vi "nav waypoint info.vi"(11 "step":i32) -> (0 "target y":i32, 1 "target x":i32, 2 "load":i32, 3 "stacking height":dbl, 4 "steps":i32)   [LabVIEW 2014]
uses:
  <vilib>/Rock Robotics/Network Tables/SD Read Boolean Array.vi
  Robot Global Data.vi
panel:
  out "Button States":bool[](array[boolean])
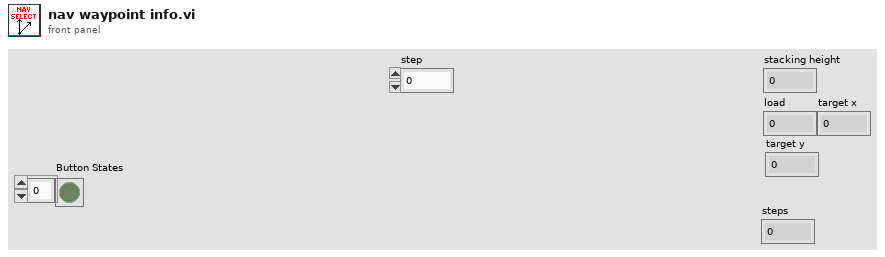
[diagram p1: front panel]
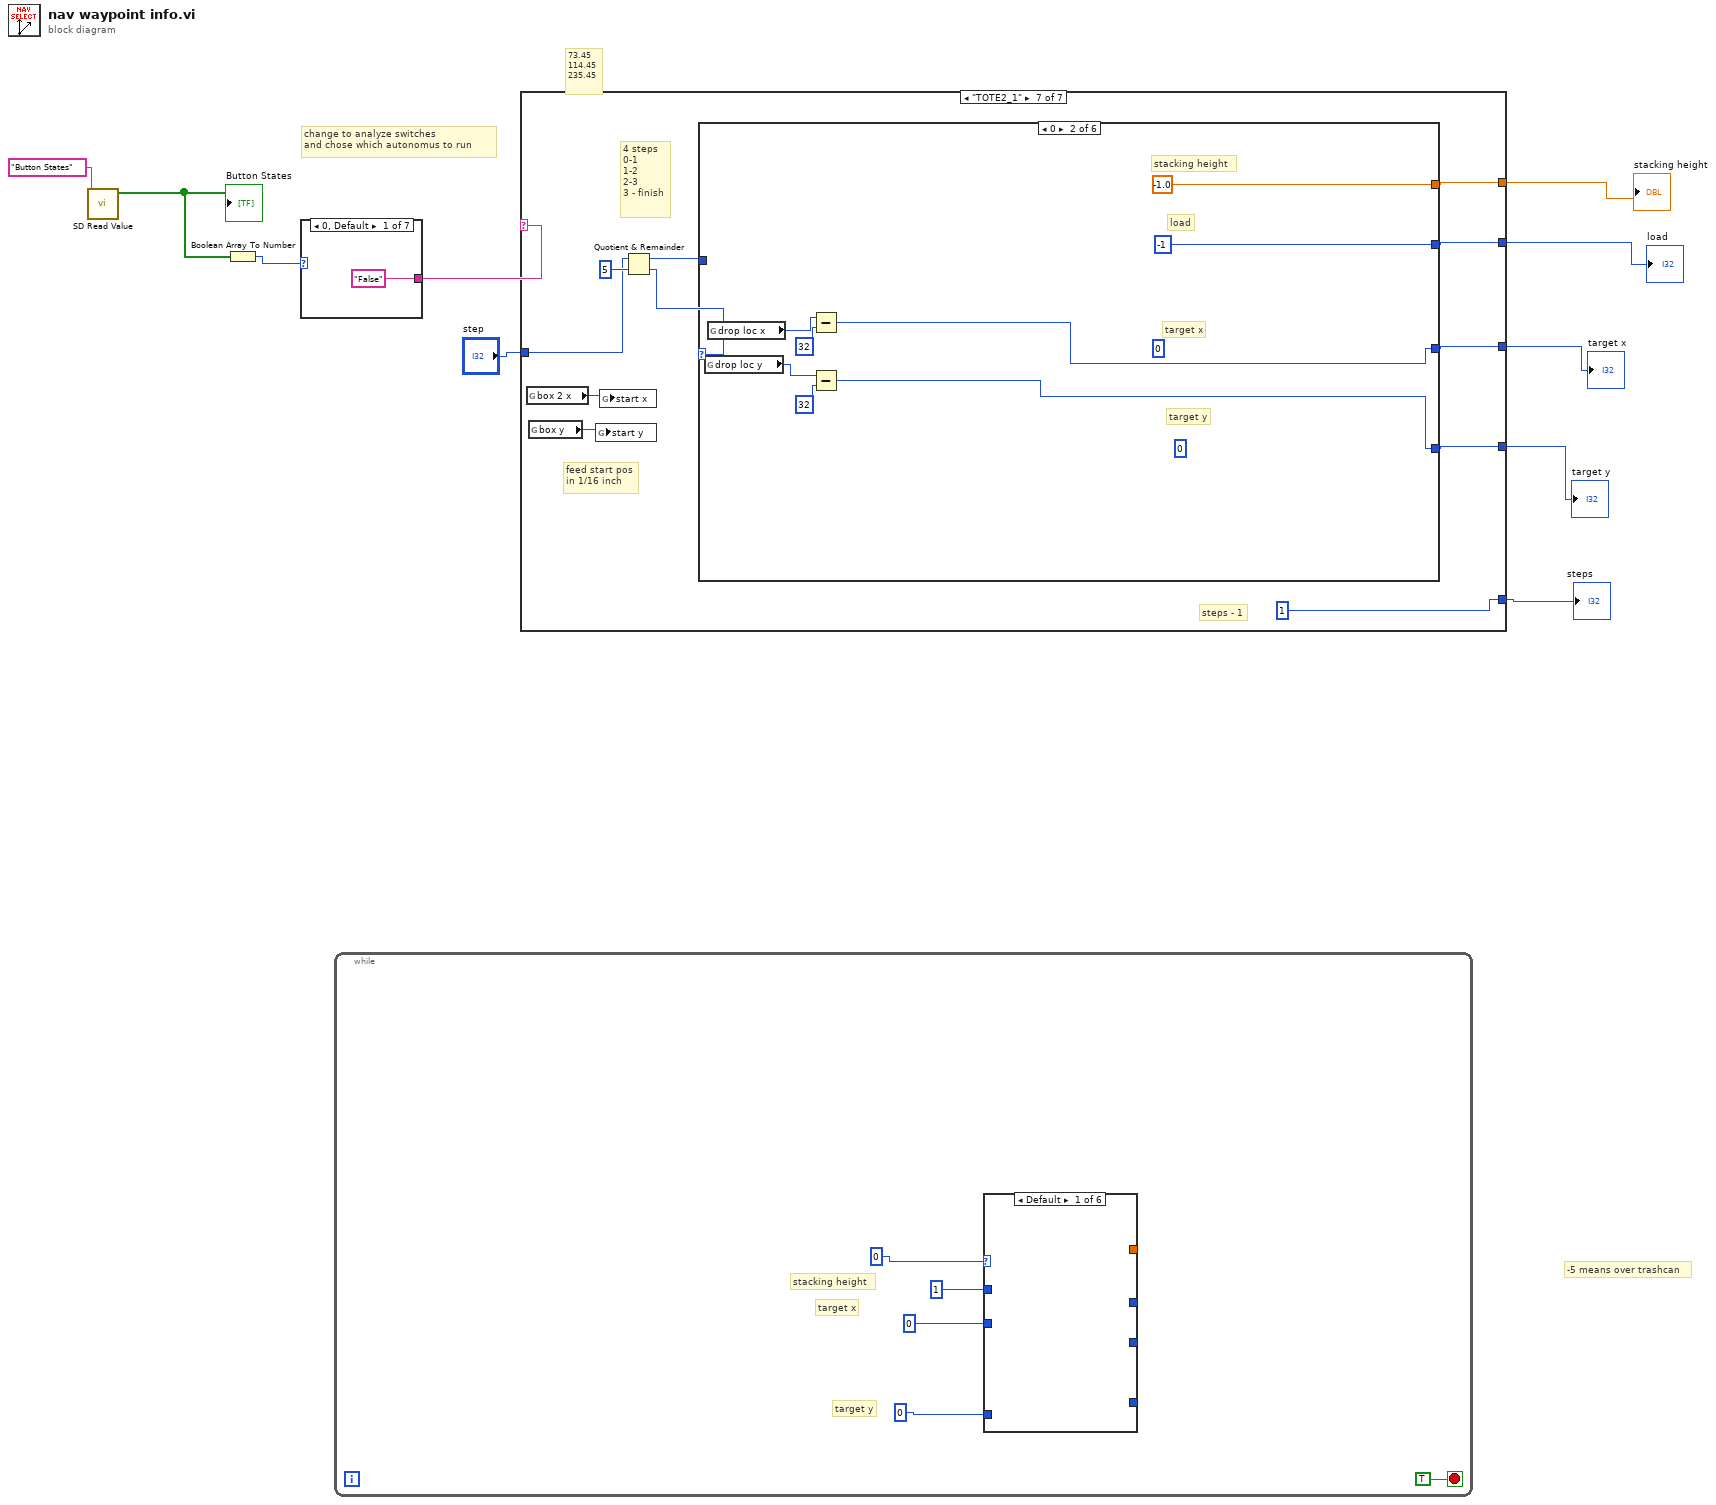
[diagram p0: block diagram]
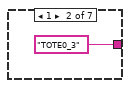
[diagram p2: hidden frame]
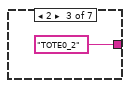
[diagram p3: hidden frame]
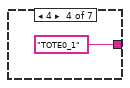
[diagram p4: hidden frame]
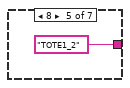
[diagram p5: hidden frame]
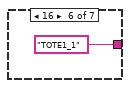
[diagram p6: hidden frame]
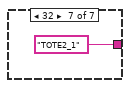
[diagram p7: hidden frame]
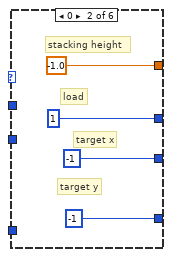
[diagram p8: hidden frame]
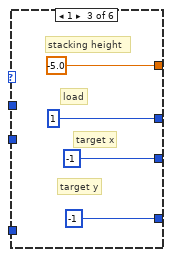
[diagram p9: hidden frame]
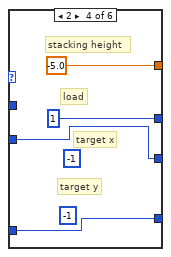
[diagram p10: hidden frame]
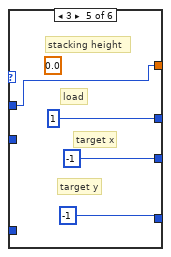
[diagram p11: hidden frame]
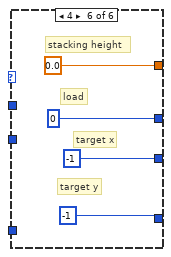
[diagram p12: hidden frame]
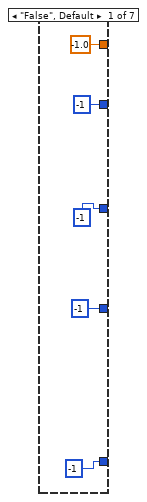
[diagram p13: hidden frame]
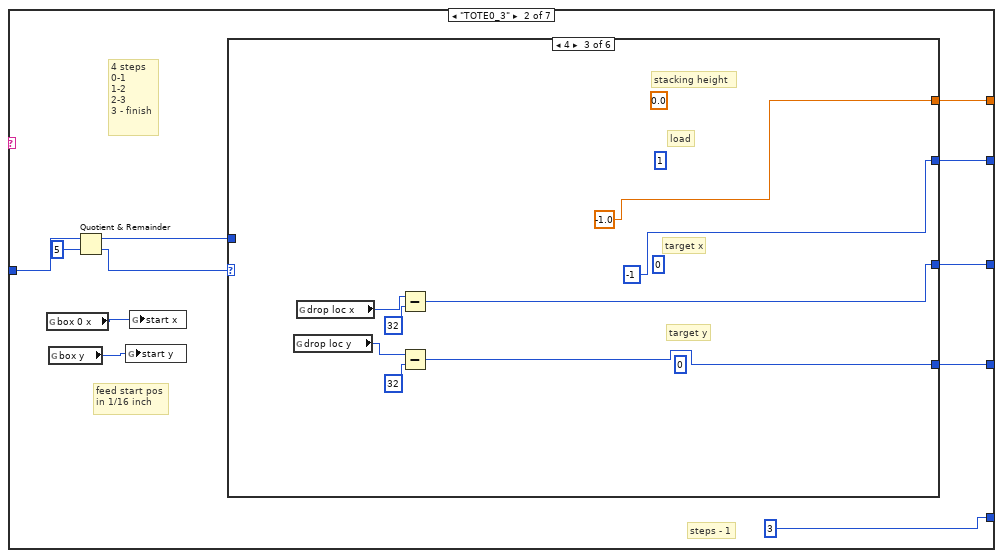
[diagram p14: hidden frame]
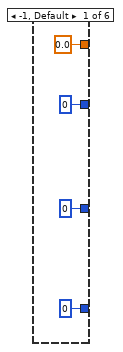
[diagram p15: hidden frame]
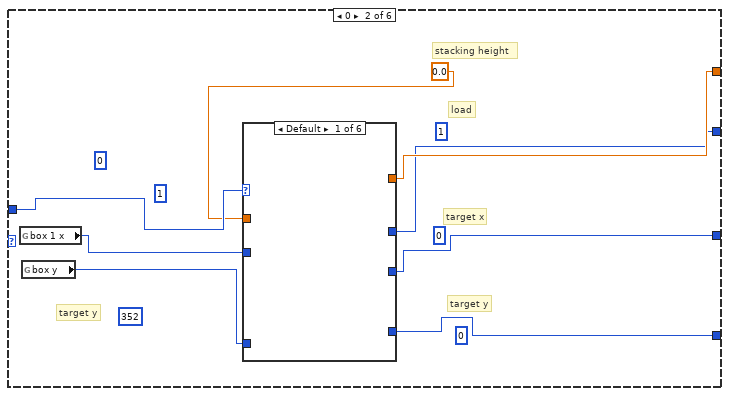
[diagram p16: hidden frame]
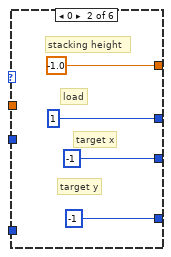
[diagram p17: hidden frame]
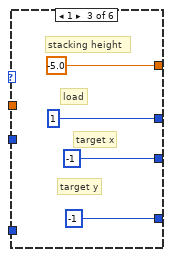
[diagram p18: hidden frame]
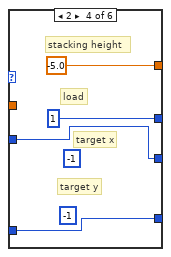
[diagram p19: hidden frame]
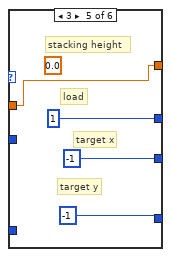
[diagram p20: hidden frame]
diagram:
  # "73.45\n114.45\n235.45"
  # "-5 means over trashcan"
  # "change to analyze switches\nand chose which autonomus to run"
  n1 = call-poly <vilib>:"SD Read Value.vi"("Name"="Button States") -> ("Boolean Array"=w3:bool[])  [unwired: 8 in, 2 out]
  "Button States" <- w3
  n2 = Boolean Array To Number(Boolean array=w3) -> (number=w2:u32)
  n3 = case shown="0, Default" w2 {
    tunnel: ["False" "TOTE0_3" "TOTE0_2" "TOTE0_1" "TOTE1_2" "TOTE1_1" "TOTE2_1"] -> w1
    frame 0, Default {
    }
    frame 1 {
    }
    frame 2 {
    }
    frame 4 {
    }
    frame 8 {
    }
    frame 16 {
    }
    frame 32 {
    }
  }
  n4 = while {
    stop <- TRUE stop-if-true
    # "target y"
    # "target x"
    # "stacking height"
    n5 = case shown="Default" 0 {
      tunnel: [_ -1.0 -5.0 -5.0 w35 0.0] -> _
      tunnel: [_ 1 1 1 1 0] -> _
      tunnel: [_ -1 -1 w34 -1 -1] -> _
      tunnel: [_ -1 -1 w33 -1 -1] -> _
      tunnel: 0 -> [_ _ _ w34 _ _]
      tunnel: 0 -> [_ _ _ w33 _ _]
      tunnel: 1 -> [_ _ _ _ w35 _]
      frame Default {
      }
      frame 0 {
        # "target y"
        # "target x"
        # "load"
        # "stacking height"
      }
      frame 1 {
        # "target y"
        # "target x"
        # "load"
        # "stacking height"
      }
      frame 2 {
        (unwired) -1
        (unwired) -1
        # "target y"
        # "target x"
        # "load"
        # "stacking height"
      }
      frame 3 {
        (unwired) 0.0
        # "target y"
        # "target x"
        # "load"
        # "stacking height"
      }
      frame 4 {
        # "target y"
        # "target x"
        # "load"
        # "stacking height"
      }
    }
  }
  n6 = case shown="\"TOTE2_1\"" w1 {
    tunnel: "step" -> [_ w53 w186 w322 w455 w596 w726]
    tunnel: [-1.0 w58 w193 w328 w463 w590 w732] -> w9
    tunnel: [-1 w57 w192 w327 w462 w591 w731] -> w8
    tunnel: [-1 w56 w191 w326 w461 w592 w730] -> w7
    tunnel: [-1 w55 w190 w325 w460 w593 w729] -> w6
    tunnel: [-1 3 2 1 2 1 1] -> w5
    frame "False", Default {
    }
    frame "TOTE0_3" {
      # "feed start pos\nin 1/16 inch"
      # "steps - 1"
      # "4 steps\n0-1\n1-2\n2-3\n3 - finish"
      n7 = global read "Robot Global Data.vi" "box 0 x"() -> (w49:i16)
      n8 = global read "Robot Global Data.vi" "box y"() -> (w48:i16)
      n9 = Quotient & Remainder(x=w53, y=5) -> (x-y*floor(x/y)=w50:i32, floor(x/y)=w51:i32)
      n10 = global write "Robot Global Data.vi" "start y"(w48) -> ()
      n11 = global write "Robot Global Data.vi" "start x"(w49) -> ()
      n12 = case shown="4" w51 {
        tunnel: [0.0 w66 -1.0 w106 w133 w160] -> w58
        tunnel: [0 w65 -1 w103 w132 w159] -> w57
        tunnel: [0 w67 w92 w102 w131 w157] -> w56
        tunnel: [0 w68 w91 w101 w130 w158] -> w55
        tunnel: w50 -> [_ w70 _ w104 w129 w162]
        frame -1, Default {
        }
        frame 0 {
          (unwired) 1
          (unwired) 352
          (unwired) 0
          (unwired) 0
          (unwired) 0
          (unwired) 1
          # "target y"
          # "target y"
          # "target x"
          # "load"
          # "stacking height"
          n13 = global read "Robot Global Data.vi" "box 1 x"() -> (w64:i16)
          n14 = global read "Robot Global Data.vi" "box y"() -> (w63:i16)
          n15 = case shown="Default" w70 {
            tunnel: [_ -1.0 -5.0 -5.0 w83 0.0] -> w66
            tunnel: [_ 1 1 1 1 0] -> w65
            tunnel: [_ -1 -1 w82 -1 -1] -> w67
            tunnel: [_ -1 -1 w81 -1 -1] -> w68
            tunnel: w64 -> [_ _ _ w82 _ _]
            tunnel: w63 -> [_ _ _ w81 _ _]
            tunnel: 0.0 -> [_ _ _ _ w83 _]
            frame Default {
            }
            frame 0 {
              # "target y"
              # "target x"
              # "load"
              # "stacking height"
            }
            frame 1 {
              # "target y"
              # "target x"
              # "load"
              # "stacking height"
            }
            frame 2 {
              (unwired) -1
              (unwired) -1
              # "target y"
              # "target x"
              # "load"
              # "stacking height"
            }
            frame 3 {
              (unwired) 0.0
              # "target y"
              # "target x"
              # "load"
              # "stacking height"
            }
            frame 4 {
              # "target y"
              # "target x"
              # "load"
              # "stacking height"
            }
          }
        }
        frame 4 {
          (unwired) 0
          (unwired) 0
          (unwired) 1
          (unwired) 0.0
          # "target y"
          # "target x"
          # "load"
          # "stacking height"
          n16 = global read "Robot Global Data.vi" "drop loc y"() -> (w93:i16)
          n17 = global read "Robot Global Data.vi" "drop loc x"() -> (w96:i16)
          n18 = Subtract(x=w96, y=i16 32) -> (x-y=w92:i16)
          n19 = Subtract(x=w93, y=i16 32) -> (x-y=w91:i16)
        }
        frame 1 {
          (unwired) 0
          (unwired) 0
          (unwired) 1
          # "target y"
          # "target x"
          # "load"
          # "stacking height inchs"
          n20 = global read "Robot Global Data.vi" "box 2 x"() -> (w99:i16)
          n21 = global read "Robot Global Data.vi" "box y"() -> (w100:i16)
          n22 = case shown="Default" w104 {
            tunnel: [_ -1.0 -5.0 -5.0 w119 0.0] -> w106
            tunnel: [_ 1 1 1 1 0] -> w103
            tunnel: [_ -1 -1 w118 -1 -1] -> w102
            tunnel: [_ -1 -1 w117 -1 -1] -> w101
            tunnel: w99 -> [_ _ _ w118 _ _]
            tunnel: w100 -> [_ _ _ w117 _ _]
            tunnel: 12.1 -> [_ _ _ _ w119 _]
            frame Default {
            }
            frame 0 {
              # "target y"
              # "target x"
              # "load"
              # "stacking height"
            }
            frame 1 {
              # "target y"
              # "target x"
              # "load"
              # "stacking height"
            }
            frame 2 {
              (unwired) -1
              (unwired) -1
              # "target y"
              # "target x"
              # "load"
              # "stacking height"
            }
            frame 3 {
              (unwired) 0.0
              # "target y"
              # "target x"
              # "load"
              # "stacking height"
            }
            frame 4 {
              # "target y"
              # "target x"
              # "load"
              # "stacking height"
            }
          }
        }
        frame 2 {
          (unwired) 0
          (unwired) 0
          (unwired) 1
          # "to box 3"
          # "target y"
          # "target x"
          # "load"
          # "stacking height inchs"
          n23 = global read "Robot Global Data.vi" "box 2 x"() -> (w128:i16)
          n24 = global read "Robot Global Data.vi" "box y"() -> (w127:i16)
          n25 = case shown="Default" w129 {
            tunnel: [_ -1.0 -5.0 -5.0 w147 0.0] -> w133
            tunnel: [_ 1 1 1 1 0] -> w132
            tunnel: [_ -1 -1 w146 -1 -1] -> w131
            tunnel: [_ -1 -1 w145 -1 -1] -> w130
            tunnel: w128 -> [_ _ _ w146 _ _]
            tunnel: w127 -> [_ _ _ w145 _ _]
            tunnel: 24.2 -> [_ _ _ _ w147 _]
            frame Default {
            }
            frame 0 {
              # "target y"
              # "target x"
              # "load"
              # "stacking height"
            }
            frame 1 {
              # "target y"
              # "target x"
              # "load"
              # "stacking height"
            }
            frame 2 {
              (unwired) -1
              (unwired) -1
              # "target y"
              # "target x"
              # "load"
              # "stacking height"
            }
            frame 3 {
              (unwired) 0.0
              # "target y"
              # "target x"
              # "load"
              # "stacking height"
            }
            frame 4 {
              # "target y"
              # "target x"
              # "load"
              # "stacking height"
            }
          }
        }
        frame 3 {
          (unwired) 0
          (unwired) 0
          (unwired) 0
          # "steps"
          # "target y"
          # "target x"
          # "load"
          # "stacking height inchs"
          n26 = global read "Robot Global Data.vi" "drop loc y"() -> (w155:i16)
          n27 = global read "Robot Global Data.vi" "drop loc x"() -> (w156:i16)
          n28 = case shown="4" w162 {
            tunnel: [_ -1.0 -5.0 -5.0 w175 0.0] -> w160
            tunnel: [_ 1 1 1 1 0] -> w159
            tunnel: [_ -1 -1 w174 -1 -1] -> w157
            tunnel: [_ -1 -1 w173 -1 -1] -> w158
            tunnel: w156 -> [_ _ _ w174 _ _]
            tunnel: w155 -> [_ _ _ w173 _ _]
            tunnel: 4.0 -> [_ _ _ _ w175 _]
            frame Default {
            }
            frame 0 {
              # "target y"
              # "target x"
              # "load"
              # "stacking height"
            }
            frame 1 {
              # "target y"
              # "target x"
              # "load"
              # "stacking height"
            }
            frame 2 {
              (unwired) -1
              (unwired) -1
              # "target y"
              # "target x"
              # "load"
              # "stacking height"
            }
            frame 3 {
              (unwired) 0.0
              # "target y"
              # "target x"
              # "load"
              # "stacking height"
            }
            frame 4 {
              # "target y"
              # "target x"
              # "load"
              # "stacking height"
            }
          }
        }
      }
    }
    frame "TOTE0_2" {
      # "feed start pos\nin 1/16 inch"
      # "steps - 1"
      # "4 steps\n0-1\n1-2\n2-3\n3 - finish"
      n29 = global read "Robot Global Data.vi" "box 0 x"() -> (w183:i16)
      n30 = global read "Robot Global Data.vi" "box y"() -> (w184:i16)
      n31 = Quotient & Remainder(x=w186, y=5) -> (x-y*floor(x/y)=w187:i32, floor(x/y)=w185:i32)
      n32 = global write "Robot Global Data.vi" "start y"(w184) -> ()
      n33 = global write "Robot Global Data.vi" "start x"(w183) -> ()
      n34 = case shown="2" w185 {
        tunnel: [0.0 w204 w232 w260 -1.0 w295] -> w193
        tunnel: [0 w203 w231 w259 -1 w294] -> w192
        tunnel: [0 w201 w230 w258 w284 w291] -> w191
        tunnel: [0 w202 w229 w257 w285 w290] -> w190
        tunnel: w187 -> [_ w200 w228 w256 _ w296]
        frame -1, Default {
        }
        frame 0 {
          (unwired) 0
          (unwired) 0
          (unwired) 0
          # "target y"
          # "target x"
          # "load"
          # "stacking height"
          n35 = global read "Robot Global Data.vi" "box 2 x"() -> (w199:i16)
          n36 = global read "Robot Global Data.vi" "box y"() -> (w198:i16)
          n37 = case shown="Default" w200 {
            tunnel: [_ -1.0 -5.0 -5.0 w218 0.0] -> w204
            tunnel: [_ 1 1 1 1 0] -> w203
            tunnel: [_ -1 -1 w217 -1 -1] -> w201
            tunnel: [_ -1 -1 w216 -1 -1] -> w202
            tunnel: w199 -> [_ _ _ w217 _ _]
            tunnel: w198 -> [_ _ _ w216 _ _]
            tunnel: 0.0 -> [_ _ _ _ w218 _]
            frame Default {
            }
            frame 0 {
              # "target y"
              # "target x"
              # "load"
              # "stacking height"
            }
            frame 1 {
              # "target y"
              # "target x"
              # "load"
              # "stacking height"
            }
            frame 2 {
              (unwired) -1
              (unwired) -1
              # "target y"
              # "target x"
              # "load"
              # "stacking height"
            }
            frame 3 {
              (unwired) 0.0
              # "target y"
              # "target x"
              # "load"
              # "stacking height"
            }
            frame 4 {
              # "target y"
              # "target x"
              # "load"
              # "stacking height"
            }
          }
        }
        frame 4 {
          (unwired) 0
          (unwired) 0
          (unwired) 1
          # "target y"
          # "target x"
          # "load"
          # "stacking height"
          n38 = global read "Robot Global Data.vi" "box 0 x"() -> (w227:i16)
          n39 = global read "Robot Global Data.vi" "box y"() -> (w226:i16)
          n40 = case shown="Default" w228 {
            tunnel: [_ -1.0 -5.0 -5.0 w246 0.0] -> w232
            tunnel: [_ 1 1 1 1 0] -> w231
            tunnel: [_ -1 -1 w245 -1 -1] -> w230
            tunnel: [_ -1 -1 w244 -1 -1] -> w229
            tunnel: w227 -> [_ _ _ w245 _ _]
            tunnel: w226 -> [_ _ _ w244 _ _]
            tunnel: 0.0 -> [_ _ _ _ w246 _]
            frame Default {
            }
            frame 0 {
              # "target y"
              # "target x"
              # "load"
              # "stacking height"
            }
            frame 1 {
              # "target y"
              # "target x"
              # "load"
              # "stacking height"
            }
            frame 2 {
              (unwired) -1
              (unwired) -1
              # "target y"
              # "target x"
              # "load"
              # "stacking height"
            }
            frame 3 {
              (unwired) 0.0
              # "target y"
              # "target x"
              # "load"
              # "stacking height"
            }
            frame 4 {
              # "target y"
              # "target x"
              # "load"
              # "stacking height"
            }
          }
        }
        frame 1 {
          (unwired) 0
          (unwired) 0
          (unwired) 1
          # "target y"
          # "target x"
          # "load"
          # "stacking height inchs"
          n41 = global read "Robot Global Data.vi" "drop loc y"() -> (w254:i16)
          n42 = global read "Robot Global Data.vi" "drop loc x"() -> (w255:i16)
          n43 = case shown="Default" w256 {
            tunnel: [_ -1.0 -5.0 -5.0 w274 0.0] -> w260
            tunnel: [_ 1 1 1 1 0] -> w259
            tunnel: [_ -1 -1 w273 -1 -1] -> w258
            tunnel: [_ -1 -1 w272 -1 -1] -> w257
            tunnel: w255 -> [_ _ _ w273 _ _]
            tunnel: w254 -> [_ _ _ w272 _ _]
            tunnel: 12.1 -> [_ _ _ _ w274 _]
            frame Default {
            }
            frame 0 {
              # "target y"
              # "target x"
              # "load"
              # "stacking height"
            }
            frame 1 {
              # "target y"
              # "target x"
              # "load"
              # "stacking height"
            }
            frame 2 {
              (unwired) -1
              (unwired) -1
              # "target y"
              # "target x"
              # "load"
              # "stacking height"
            }
            frame 3 {
              (unwired) 0.0
              # "target y"
              # "target x"
              # "load"
              # "stacking height"
            }
            frame 4 {
              # "target y"
              # "target x"
              # "load"
              # "stacking height"
            }
          }
        }
        frame 2 {
          (unwired) 0
          (unwired) 0
          # "target y"
          # "target x"
          # "load"
          # "stacking height inchs"
          n44 = global read "Robot Global Data.vi" "drop loc y"() -> (w286:i16)
          n45 = global read "Robot Global Data.vi" "drop loc x"() -> (w289:i16)
          n46 = Subtract(x=w289, y=i16 32) -> (x-y=w284:i16)
          n47 = Subtract(x=w286, y=i16 32) -> (x-y=w285:i16)
        }
        frame 3 {
          (unwired) 0
          # "steps"
          # "target y"
          # "target x"
          # "load"
          # "stacking height inchs"
          n48 = case shown="Default" w296 {
            tunnel: [_ -1.0 -5.0 -5.0 w310 0.0] -> w295
            tunnel: [_ 1 1 1 1 0] -> w294
            tunnel: [_ -1 -1 w309 -1 -1] -> w291
            tunnel: [_ -1 -1 w308 -1 -1] -> w290
            tunnel: 0 -> [_ _ _ w309 _ _]
            tunnel: 0 -> [_ _ _ w308 _ _]
            tunnel: 4.0 -> [_ _ _ _ w310 _]
            frame Default {
            }
            frame 0 {
              # "target y"
              # "target x"
              # "load"
              # "stacking height"
            }
            frame 1 {
              # "target y"
              # "target x"
              # "load"
              # "stacking height"
            }
            frame 2 {
              (unwired) -1
              (unwired) -1
              # "target y"
              # "target x"
              # "load"
              # "stacking height"
            }
            frame 3 {
              (unwired) 0.0
              # "target y"
              # "target x"
              # "load"
              # "stacking height"
            }
            frame 4 {
              # "target y"
              # "target x"
              # "load"
              # "stacking height"
            }
          }
        }
      }
    }
    frame "TOTE0_1" {
      # "feed start pos\nin 1/16 inch"
      # "steps - 1"
      # "4 steps\n0-1\n1-2\n2-3\n3 - finish"
      n49 = global read "Robot Global Data.vi" "box 0 x"() -> (w319:i16)
      n50 = global read "Robot Global Data.vi" "box y"() -> (w318:i16)
      n51 = global write "Robot Global Data.vi" "start y"(w318) -> ()
      n52 = global write "Robot Global Data.vi" "start x"(w319) -> ()
      n53 = Quotient & Remainder(x=w322, y=5) -> (x-y*floor(x/y)=w321:i32, floor(x/y)=w320:i32)
      n54 = case shown="1" w320 {
        tunnel: [0.0 w339 w368 -1.0 w402 w432] -> w328
        tunnel: [0 w338 w366 -1 w401 w431] -> w327
        tunnel: [0 w337 w363 w392 w398 w428] -> w326
        tunnel: [0 w336 w362 w391 w397 w427] -> w325
        tunnel: w321 -> [_ w335 w361 _ w403 w425]
        frame -1, Default {
        }
        frame 0 {
          (unwired) 0
          (unwired) 0
          (unwired) 1
          # "target y"
          # "target x"
          # "load"
          # "stacking height"
          n55 = global read "Robot Global Data.vi" "drop loc y"() -> (w333:i16)
          n56 = global read "Robot Global Data.vi" "drop loc x"() -> (w334:i16)
          n57 = case shown="Default" w335 {
            tunnel: [_ -1.0 -5.0 -5.0 w353 0.0] -> w339
            tunnel: [_ 1 1 1 1 0] -> w338
            tunnel: [_ -1 -1 w352 -1 -1] -> w337
            tunnel: [_ -1 -1 w351 -1 -1] -> w336
            tunnel: w334 -> [_ _ _ w352 _ _]
            tunnel: w333 -> [_ _ _ w351 _ _]
            tunnel: 0.0 -> [_ _ _ _ w353 _]
            frame Default {
            }
            frame 0 {
              # "target y"
              # "target x"
              # "load"
              # "stacking height"
            }
            frame 1 {
              # "target y"
              # "target x"
              # "load"
              # "stacking height"
            }
            frame 2 {
              (unwired) -1
              (unwired) -1
              # "target y"
              # "target x"
              # "load"
              # "stacking height"
            }
            frame 3 {
              (unwired) 0.0
              # "target y"
              # "target x"
              # "load"
              # "stacking height"
            }
            frame 4 {
              # "target y"
              # "target x"
              # "load"
              # "stacking height"
            }
          }
        }
        frame 4 {
          (unwired) 1
          # "target y"
          # "target x"
          # "load"
          # "stacking height"
          n58 = case shown="Default" w361 {
            tunnel: [_ -1.0 -5.0 -5.0 w381 0.0] -> w368
            tunnel: [_ 1 1 1 1 0] -> w366
            tunnel: [_ -1 -1 w380 -1 -1] -> w363
            tunnel: [_ -1 -1 w379 -1 -1] -> w362
            tunnel: 0 -> [_ _ _ w380 _ _]
            tunnel: 0 -> [_ _ _ w379 _ _]
            tunnel: 0.0 -> [_ _ _ _ w381 _]
            frame Default {
            }
            frame 0 {
              # "target y"
              # "target x"
              # "load"
              # "stacking height"
            }
            frame 1 {
              # "target y"
              # "target x"
              # "load"
              # "stacking height"
            }
            frame 2 {
              (unwired) -1
              (unwired) -1
              # "target y"
              # "target x"
              # "load"
              # "stacking height"
            }
            frame 3 {
              (unwired) 0.0
              # "target y"
              # "target x"
              # "load"
              # "stacking height"
            }
            frame 4 {
              # "target y"
              # "target x"
              # "load"
              # "stacking height"
            }
          }
        }
        frame 1 {
          (unwired) 0
          (unwired) 0
          # "target y"
          # "target x"
          # "load"
          # "stacking height inchs"
          n59 = global read "Robot Global Data.vi" "drop loc y"() -> (w393:i16)
          n60 = global read "Robot Global Data.vi" "drop loc x"() -> (w396:i16)
          n61 = Subtract(x=w396, y=i16 32) -> (x-y=w392:i16)
          n62 = Subtract(x=w393, y=i16 32) -> (x-y=w391:i16)
        }
        frame 2 {
          (unwired) 1
          # "target y"
          # "target x"
          # "load"
          # "stacking height inchs"
          n63 = case shown="Default" w403 {
            tunnel: [_ -1.0 -5.0 -5.0 w417 0.0] -> w402
            tunnel: [_ 1 1 1 1 0] -> w401
            tunnel: [_ -1 -1 w416 -1 -1] -> w398
            tunnel: [_ -1 -1 w415 -1 -1] -> w397
            tunnel: 0 -> [_ _ _ w416 _ _]
            tunnel: 0 -> [_ _ _ w415 _ _]
            tunnel: 24.2 -> [_ _ _ _ w417 _]
            frame Default {
            }
            frame 0 {
              # "target y"
              # "target x"
              # "load"
              # "stacking height"
            }
            frame 1 {
              # "target y"
              # "target x"
              # "load"
              # "stacking height"
            }
            frame 2 {
              (unwired) -1
              (unwired) -1
              # "target y"
              # "target x"
              # "load"
              # "stacking height"
            }
            frame 3 {
              (unwired) 0.0
              # "target y"
              # "target x"
              # "load"
              # "stacking height"
            }
            frame 4 {
              # "target y"
              # "target x"
              # "load"
              # "stacking height"
            }
          }
        }
        frame 3 {
          (unwired) 0
          # "steps"
          # "target y"
          # "target x"
          # "load"
          # "stacking height inchs"
          n64 = case shown="Default" w425 {
            tunnel: [_ -1.0 -5.0 -5.0 w445 0.0] -> w432
            tunnel: [_ 1 1 1 1 0] -> w431
            tunnel: [_ -1 -1 w444 -1 -1] -> w428
            tunnel: [_ -1 -1 w443 -1 -1] -> w427
            tunnel: 0 -> [_ _ _ w444 _ _]
            tunnel: 0 -> [_ _ _ w443 _ _]
            tunnel: 4.0 -> [_ _ _ _ w445 _]
            frame Default {
            }
            frame 0 {
              # "target y"
              # "target x"
              # "load"
              # "stacking height"
            }
            frame 1 {
              # "target y"
              # "target x"
              # "load"
              # "stacking height"
            }
            frame 2 {
              (unwired) -1
              (unwired) -1
              # "target y"
              # "target x"
              # "load"
              # "stacking height"
            }
            frame 3 {
              (unwired) 0.0
              # "target y"
              # "target x"
              # "load"
              # "stacking height"
            }
            frame 4 {
              # "target y"
              # "target x"
              # "load"
              # "stacking height"
            }
          }
        }
      }
    }
    frame "TOTE1_2" {
      # "feed start pos\nin 1/16 inch"
      # "steps - 1"
      # "4 steps\n0-1\n1-2\n2-3\n3 - finish"
      n65 = global read "Robot Global Data.vi" "box 1 x"() -> (w454:i16)
      n66 = global read "Robot Global Data.vi" "box y"() -> (w453:i16)
      n67 = Quotient & Remainder(x=w455, y=5) -> (x-y*floor(x/y)=w457:i32, floor(x/y)=w456:i32)
      n68 = global write "Robot Global Data.vi" "start y"(w453) -> ()
      n69 = global write "Robot Global Data.vi" "start x"(w454) -> ()
      n70 = case shown="2" w456 {
        tunnel: [0.0 w473 w501 w529 -1.0 w567] -> w463
        tunnel: [0 w472 w500 w528 -1 w564] -> w462
        tunnel: [0 w471 w497 w526 w555 w561] -> w461
        tunnel: [0 w470 w496 w527 w554 w560] -> w460
        tunnel: w457 -> [_ w475 w502 w530 _ w565]
        frame -1, Default {
        }
        frame 0 {
          (unwired) 0
          (unwired) 0
          (unwired) 1
          # "target y"
          # "target x"
          # "load"
          # "stacking height"
          n71 = global read "Robot Global Data.vi" "box 2 x"() -> (w469:i16)
          n72 = global read "Robot Global Data.vi" "box y"() -> (w468:i16)
          n73 = case shown="Default" w475 {
            tunnel: [_ -1.0 -5.0 -5.0 w488 0.0] -> w473
            tunnel: [_ 1 1 1 1 0] -> w472
            tunnel: [_ -1 -1 w487 -1 -1] -> w471
            tunnel: [_ -1 -1 w486 -1 -1] -> w470
            tunnel: w469 -> [_ _ _ w487 _ _]
            tunnel: w468 -> [_ _ _ w486 _ _]
            tunnel: 0.0 -> [_ _ _ _ w488 _]
            frame Default {
            }
            frame 0 {
              # "target y"
              # "target x"
              # "load"
              # "stacking height"
            }
            frame 1 {
              # "target y"
              # "target x"
              # "load"
              # "stacking height"
            }
            frame 2 {
              (unwired) -1
              (unwired) -1
              # "target y"
              # "target x"
              # "load"
              # "stacking height"
            }
            frame 3 {
              (unwired) 0.0
              # "target y"
              # "target x"
              # "load"
              # "stacking height"
            }
            frame 4 {
              # "target y"
              # "target x"
              # "load"
              # "stacking height"
            }
          }
        }
        frame 4 {
          (unwired) 1
          # "target y"
          # "target x"
          # "load"
          # "stacking height"
          n74 = case shown="Default" w502 {
            tunnel: [_ -1.0 -5.0 -5.0 w516 0.0] -> w501
            tunnel: [_ 1 1 1 1 0] -> w500
            tunnel: [_ -1 -1 w515 -1 -1] -> w497
            tunnel: [_ -1 -1 w514 -1 -1] -> w496
            tunnel: 0 -> [_ _ _ w515 _ _]
            tunnel: 0 -> [_ _ _ w514 _ _]
            tunnel: 0.0 -> [_ _ _ _ w516 _]
            frame Default {
            }
            frame 0 {
              # "target y"
              # "target x"
              # "load"
              # "stacking height"
            }
            frame 1 {
              # "target y"
              # "target x"
              # "load"
              # "stacking height"
            }
            frame 2 {
              (unwired) -1
              (unwired) -1
              # "target y"
              # "target x"
              # "load"
              # "stacking height"
            }
            frame 3 {
              (unwired) 0.0
              # "target y"
              # "target x"
              # "load"
              # "stacking height"
            }
            frame 4 {
              # "target y"
              # "target x"
              # "load"
              # "stacking height"
            }
          }
        }
        frame 1 {
          (unwired) 0
          (unwired) 0
          (unwired) 1
          # "target y"
          # "target x"
          # "load"
          # "stacking height inchs"
          n75 = global read "Robot Global Data.vi" "drop loc y"() -> (w524:i16)
          n76 = global read "Robot Global Data.vi" "drop loc x"() -> (w525:i16)
          n77 = case shown="Default" w530 {
            tunnel: [_ -1.0 -5.0 -5.0 w544 0.0] -> w529
            tunnel: [_ 1 1 1 1 0] -> w528
            tunnel: [_ -1 -1 w543 -1 -1] -> w526
            tunnel: [_ -1 -1 w542 -1 -1] -> w527
            tunnel: w525 -> [_ _ _ w543 _ _]
            tunnel: w524 -> [_ _ _ w542 _ _]
            tunnel: 0.0 -> [_ _ _ _ w544 _]
            frame Default {
            }
            frame 0 {
              # "target y"
              # "target x"
              # "load"
              # "stacking height"
            }
            frame 1 {
              # "target y"
              # "target x"
              # "load"
              # "stacking height"
            }
            frame 2 {
              (unwired) -1
              (unwired) -1
              # "target y"
              # "target x"
              # "load"
              # "stacking height"
            }
            frame 3 {
              (unwired) 0.0
              # "target y"
              # "target x"
              # "load"
              # "stacking height"
            }
            frame 4 {
              # "target y"
              # "target x"
              # "load"
              # "stacking height"
            }
          }
        }
        frame 2 {
          (unwired) 0
          (unwired) 0
          # "target y"
          # "target x"
          # "load"
          # "stacking height inchs"
          n78 = global read "Robot Global Data.vi" "drop loc y"() -> (w556:i16)
          n79 = global read "Robot Global Data.vi" "drop loc x"() -> (w559:i16)
          n80 = Subtract(x=w559, y=i16 32) -> (x-y=w555:i16)
          n81 = Subtract(x=w556, y=i16 32) -> (x-y=w554:i16)
        }
        frame 3 {
          (unwired) 0
          # "steps"
          # "target y"
          # "target x"
          # "load"
          # "stacking height inchs"
          n82 = case shown="Default" w565 {
            tunnel: [_ -1.0 -5.0 -5.0 w580 0.0] -> w567
            tunnel: [_ 1 1 1 1 0] -> w564
            tunnel: [_ -1 -1 w579 -1 -1] -> w561
            tunnel: [_ -1 -1 w578 -1 -1] -> w560
            tunnel: 0 -> [_ _ _ w579 _ _]
            tunnel: 0 -> [_ _ _ w578 _ _]
            tunnel: 4.0 -> [_ _ _ _ w580 _]
            frame Default {
            }
            frame 0 {
              # "target y"
              # "target x"
              # "load"
              # "stacking height"
            }
            frame 1 {
              # "target y"
              # "target x"
              # "load"
              # "stacking height"
            }
            frame 2 {
              (unwired) -1
              (unwired) -1
              # "target y"
              # "target x"
              # "load"
              # "stacking height"
            }
            frame 3 {
              (unwired) 0.0
              # "target y"
              # "target x"
              # "load"
              # "stacking height"
            }
            frame 4 {
              # "target y"
              # "target x"
              # "load"
              # "stacking height"
            }
          }
        }
      }
    }
    frame "TOTE1_1" {
      # "feed start pos\nin 1/16 inch"
      # "steps - 1"
      # "4 steps\n0-1\n1-2\n2-3\n3 - finish"
      n83 = global read "Robot Global Data.vi" "box 1 x"() -> (w589:i16)
      n84 = global read "Robot Global Data.vi" "box y"() -> (w588:i16)
      n85 = global write "Robot Global Data.vi" "start y"(w588) -> ()
      n86 = global write "Robot Global Data.vi" "start x"(w589) -> ()
      n87 = Quotient & Remainder(x=w596, y=5) -> (x-y*floor(x/y)=w595:i32, floor(x/y)=w594:i32)
      n88 = case shown="1" w594 {
        tunnel: [0.0 w609 w637 -1.0 w673 w700] -> w590
        tunnel: [0 w608 w636 -1 w672 w699] -> w591
        tunnel: [0 w606 w635 w662 w669 w696] -> w592
        tunnel: [0 w607 w634 w661 w668 w695] -> w593
        tunnel: w595 -> [_ w605 w633 _ w667 w701]
        frame -1, Default {
        }
        frame 0 {
          (unwired) 0
          (unwired) 0
          (unwired) 0
          # "target y"
          # "target x"
          # "load"
          # "stacking height"
          n89 = global read "Robot Global Data.vi" "drop loc y"() -> (w603:i16)
          n90 = global read "Robot Global Data.vi" "drop loc x"() -> (w604:i16)
          n91 = case shown="Default" w605 {
            tunnel: [_ -1.0 -5.0 -5.0 w623 0.0] -> w609
            tunnel: [_ 1 1 1 1 0] -> w608
            tunnel: [_ -1 -1 w622 -1 -1] -> w606
            tunnel: [_ -1 -1 w621 -1 -1] -> w607
            tunnel: w604 -> [_ _ _ w622 _ _]
            tunnel: w603 -> [_ _ _ w621 _ _]
            tunnel: 0.0 -> [_ _ _ _ w623 _]
            frame Default {
            }
            frame 0 {
              # "target y"
              # "target x"
              # "load"
              # "stacking height"
            }
            frame 1 {
              # "target y"
              # "target x"
              # "load"
              # "stacking height"
            }
            frame 2 {
              (unwired) -1
              (unwired) -1
              # "target y"
              # "target x"
              # "load"
              # "stacking height"
            }
            frame 3 {
              (unwired) 0.0
              # "target y"
              # "target x"
              # "load"
              # "stacking height"
            }
            frame 4 {
              # "target y"
              # "target x"
              # "load"
              # "stacking height"
            }
          }
        }
        frame 4 {
          (unwired) 0
          (unwired) 0
          (unwired) 1
          # "target y"
          # "target x"
          # "load"
          # "stacking height"
          n92 = global read "Robot Global Data.vi" "drop loc y"() -> (w631:i16)
          n93 = global read "Robot Global Data.vi" "drop loc x"() -> (w632:i16)
          n94 = case shown="Default" w633 {
            tunnel: [_ -1.0 -5.0 -5.0 w651 0.0] -> w637
            tunnel: [_ 1 1 1 1 0] -> w636
            tunnel: [_ -1 -1 w650 -1 -1] -> w635
            tunnel: [_ -1 -1 w649 -1 -1] -> w634
            tunnel: w632 -> [_ _ _ w650 _ _]
            tunnel: w631 -> [_ _ _ w649 _ _]
            tunnel: 0.0 -> [_ _ _ _ w651 _]
            frame Default {
            }
            frame 0 {
              # "target y"
              # "target x"
              # "load"
              # "stacking height"
            }
            frame 1 {
              # "target y"
              # "target x"
              # "load"
              # "stacking height"
            }
            frame 2 {
              (unwired) -1
              (unwired) -1
              # "target y"
              # "target x"
              # "load"
              # "stacking height"
            }
            frame 3 {
              (unwired) 0.0
              # "target y"
              # "target x"
              # "load"
              # "stacking height"
            }
            frame 4 {
              # "target y"
              # "target x"
              # "load"
              # "stacking height"
            }
          }
        }
        frame 1 {
          (unwired) 0
          (unwired) 0
          # "target y"
          # "target x"
          # "load"
          # "stacking height inchs"
          n95 = global read "Robot Global Data.vi" "drop loc y"() -> (w663:i16)
          n96 = global read "Robot Global Data.vi" "drop loc x"() -> (w666:i16)
          n97 = Subtract(x=w666, y=i16 32) -> (x-y=w662:i16)
          n98 = Subtract(x=w663, y=i16 32) -> (x-y=w661:i16)
        }
        frame 2 {
          (unwired) 1
          # "target y"
          # "target x"
          # "load"
          # "stacking height inchs"
          n99 = case shown="Default" w667 {
            tunnel: [_ -1.0 -5.0 -5.0 w687 0.0] -> w673
            tunnel: [_ 1 1 1 1 0] -> w672
            tunnel: [_ -1 -1 w686 -1 -1] -> w669
            tunnel: [_ -1 -1 w685 -1 -1] -> w668
            tunnel: 0 -> [_ _ _ w686 _ _]
            tunnel: 0 -> [_ _ _ w685 _ _]
            tunnel: 24.2 -> [_ _ _ _ w687 _]
            frame Default {
            }
            frame 0 {
              # "target y"
              # "target x"
              # "load"
              # "stacking height"
            }
            frame 1 {
              # "target y"
              # "target x"
              # "load"
              # "stacking height"
            }
            frame 2 {
              (unwired) -1
              (unwired) -1
              # "target y"
              # "target x"
              # "load"
              # "stacking height"
            }
            frame 3 {
              (unwired) 0.0
              # "target y"
              # "target x"
              # "load"
              # "stacking height"
            }
            frame 4 {
              # "target y"
              # "target x"
              # "load"
              # "stacking height"
            }
          }
        }
        frame 3 {
          (unwired) 0
          # "steps"
          # "target y"
          # "target x"
          # "load"
          # "stacking height inchs"
          n100 = case shown="Default" w701 {
            tunnel: [_ -1.0 -5.0 -5.0 w715 0.0] -> w700
            tunnel: [_ 1 1 1 1 0] -> w699
            tunnel: [_ -1 -1 w714 -1 -1] -> w696
            tunnel: [_ -1 -1 w713 -1 -1] -> w695
            tunnel: 0 -> [_ _ _ w714 _ _]
            tunnel: 0 -> [_ _ _ w713 _ _]
            tunnel: 4.0 -> [_ _ _ _ w715 _]
            frame Default {
            }
            frame 0 {
              # "target y"
              # "target x"
              # "load"
              # "stacking height"
            }
            frame 1 {
              # "target y"
              # "target x"
              # "load"
              # "stacking height"
            }
            frame 2 {
              (unwired) -1
              (unwired) -1
              # "target y"
              # "target x"
              # "load"
              # "stacking height"
            }
            frame 3 {
              (unwired) 0.0
              # "target y"
              # "target x"
              # "load"
              # "stacking height"
            }
            frame 4 {
              # "target y"
              # "target x"
              # "load"
              # "stacking height"
            }
          }
        }
      }
    }
    frame "TOTE2_1" {
      # "feed start pos\nin 1/16 inch"
      # "steps - 1"
      # "4 steps\n0-1\n1-2\n2-3\n3 - finish"
      n101 = global read "Robot Global Data.vi" "box 2 x"() -> (w724:i16)
      n102 = global read "Robot Global Data.vi" "box y"() -> (w723:i16)
      n103 = global write "Robot Global Data.vi" "start y"(w723) -> ()
      n104 = global write "Robot Global Data.vi" "start x"(w724) -> ()
      n105 = Quotient & Remainder(x=w726, y=5) -> (x-y*floor(x/y)=w727:i32, floor(x/y)=w725:i32)
      n106 = case shown="0" w725 {
        tunnel: [0.0 -1.0 w752 w780 w808 w835] -> w732
        tunnel: [0 -1 w751 w779 w807 w834] -> w731
        tunnel: [0 w741 w748 w777 w804 w831] -> w730
        tunnel: [0 w740 w747 w775 w803 w830] -> w729
        tunnel: w727 -> [_ _ w746 w774 w802 w836]
        frame -1, Default {
        }
        frame 0 {
          (unwired) 0
          (unwired) 0
          # "target y"
          # "target x"
          # "load"
          # "stacking height"
          n107 = global read "Robot Global Data.vi" "drop loc y"() -> (w742:i16)
          n108 = global read "Robot Global Data.vi" "drop loc x"() -> (w745:i16)
          n109 = Subtract(x=w745, y=i16 32) -> (x-y=w741:i16)
          n110 = Subtract(x=w742, y=i16 32) -> (x-y=w740:i16)
        }
        frame 4 {
          (unwired) 1
          # "target y"
          # "target x"
          # "load"
          # "stacking height"
          n111 = case shown="Default" w746 {
            tunnel: [_ -1.0 -5.0 -5.0 w766 0.0] -> w752
            tunnel: [_ 1 1 1 1 0] -> w751
            tunnel: [_ -1 -1 w765 -1 -1] -> w748
            tunnel: [_ -1 -1 w764 -1 -1] -> w747
            tunnel: 0 -> [_ _ _ w765 _ _]
            tunnel: 0 -> [_ _ _ w764 _ _]
            tunnel: 0.0 -> [_ _ _ _ w766 _]
            frame Default {
            }
            frame 0 {
              # "target y"
              # "target x"
              # "load"
              # "stacking height"
            }
            frame 1 {
              # "target y"
              # "target x"
              # "load"
              # "stacking height"
            }
            frame 2 {
              (unwired) -1
              (unwired) -1
              # "target y"
              # "target x"
              # "load"
              # "stacking height"
            }
            frame 3 {
              (unwired) 0.0
              # "target y"
              # "target x"
              # "load"
              # "stacking height"
            }
            frame 4 {
              # "target y"
              # "target x"
              # "load"
              # "stacking height"
            }
          }
        }
        frame 1 {
          (unwired) 1
          # "target y"
          # "target x"
          # "load"
          # "stacking height inchs"
          n112 = case shown="Default" w774 {
            tunnel: [_ -1.0 -5.0 -5.0 w794 0.0] -> w780
            tunnel: [_ 1 1 1 1 0] -> w779
            tunnel: [_ -1 -1 w793 -1 -1] -> w777
            tunnel: [_ -1 -1 w792 -1 -1] -> w775
            tunnel: 0 -> [_ _ _ w793 _ _]
            tunnel: 0 -> [_ _ _ w792 _ _]
            tunnel: 12.1 -> [_ _ _ _ w794 _]
            frame Default {
            }
            frame 0 {
              # "target y"
              # "target x"
              # "load"
              # "stacking height"
            }
            frame 1 {
              # "target y"
              # "target x"
              # "load"
              # "stacking height"
            }
            frame 2 {
              (unwired) -1
              (unwired) -1
              # "target y"
              # "target x"
              # "load"
              # "stacking height"
            }
            frame 3 {
              (unwired) 0.0
              # "target y"
              # "target x"
              # "load"
              # "stacking height"
            }
            frame 4 {
              # "target y"
              # "target x"
              # "load"
              # "stacking height"
            }
          }
        }
        frame 2 {
          (unwired) 1
          # "target y"
          # "target x"
          # "load"
          # "stacking height inchs"
          n113 = case shown="Default" w802 {
            tunnel: [_ -1.0 -5.0 -5.0 w822 0.0] -> w808
            tunnel: [_ 1 1 1 1 0] -> w807
            tunnel: [_ -1 -1 w821 -1 -1] -> w804
            tunnel: [_ -1 -1 w820 -1 -1] -> w803
            tunnel: 0 -> [_ _ _ w821 _ _]
            tunnel: 0 -> [_ _ _ w820 _ _]
            tunnel: 24.2 -> [_ _ _ _ w822 _]
            frame Default {
            }
            frame 0 {
              # "target y"
              # "target x"
              # "load"
              # "stacking height"
            }
            frame 1 {
              # "target y"
              # "target x"
              # "load"
              # "stacking height"
            }
            frame 2 {
              (unwired) -1
              (unwired) -1
              # "target y"
              # "target x"
              # "load"
              # "stacking height"
            }
            frame 3 {
              (unwired) 0.0
              # "target y"
              # "target x"
              # "load"
              # "stacking height"
            }
            frame 4 {
              # "target y"
              # "target x"
              # "load"
              # "stacking height"
            }
          }
        }
        frame 3 {
          (unwired) 0
          # "steps"
          # "target y"
          # "target x"
          # "load"
          # "stacking height inchs"
          n114 = case shown="Default" w836 {
            tunnel: [_ -1.0 -5.0 -5.0 w850 0.0] -> w835
            tunnel: [_ 1 1 1 1 0] -> w834
            tunnel: [_ -1 -1 w849 -1 -1] -> w831
            tunnel: [_ -1 -1 w848 -1 -1] -> w830
            tunnel: 0 -> [_ _ _ w849 _ _]
            tunnel: 0 -> [_ _ _ w848 _ _]
            tunnel: 4.0 -> [_ _ _ _ w850 _]
            frame Default {
            }
            frame 0 {
              # "target y"
              # "target x"
              # "load"
              # "stacking height"
            }
            frame 1 {
              # "target y"
              # "target x"
              # "load"
              # "stacking height"
            }
            frame 2 {
              (unwired) -1
              (unwired) -1
              # "target y"
              # "target x"
              # "load"
              # "stacking height"
            }
            frame 3 {
              (unwired) 0.0
              # "target y"
              # "target x"
              # "load"
              # "stacking height"
            }
            frame 4 {
              # "target y"
              # "target x"
              # "load"
              # "stacking height"
            }
          }
        }
      }
    }
  }
  "load" <- w8
  "target x" <- w7
  "target y" <- w6
  "stacking height" <- w9
  "steps" <- w5
